vi "Read Mission Upload Msg.vi"(8 "error in (no error)":errorcluster, 11 "Load Mission Message in":refnum<class "Mission Upload Message.lvclass">) -> (0 "error out":errorcluster, 2 "Mission":T1[](array[typedef]) {"GPS Longitude" format="%.6g"; "GPS Latitude" format="%.6g"}, 3 "Load Mission Message out":refnum<class "Mission Upload Message.lvclass">)   [LabVIEW 2015, in "RDS Child Messages.lvlib" / "Mission Upload Message.lvclass"]
uses:
  Mission Upload Message.lvclass
  RDS Mission Controller Actor/MissionOp.ctl
  Mission Upload Message.lvclass/Mission Upload Message.ctl
  RDS Mission Controller Actor/RDS Mission Controller Actor.lvlib
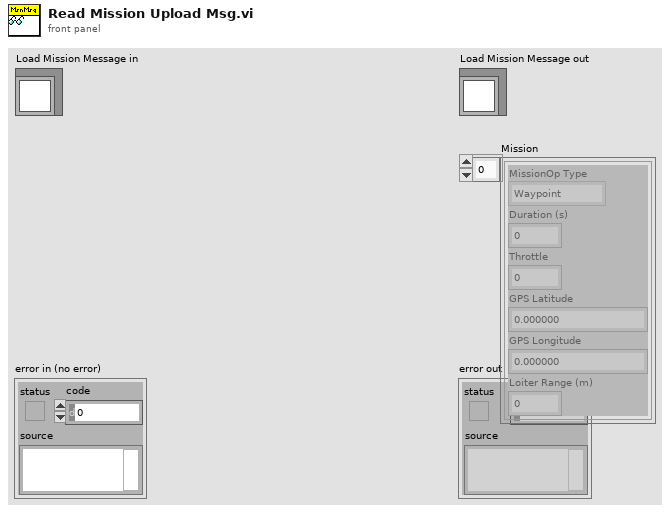
[diagram p1: front panel]
types:
  T1 = typedef "RDS Mission Controller Actor.lvlib/MissionOp.ctl" = cluster{"MissionOp Type":enum16{"Waypoint", "Loiter", "Wait", "Deploy AIP", "Stow AIP"}, "Duration (s)":u16, "Throttle":i16, "GPS Latitude":dbl, "GPS Longitude":dbl, "Loiter Range (m)":u16}
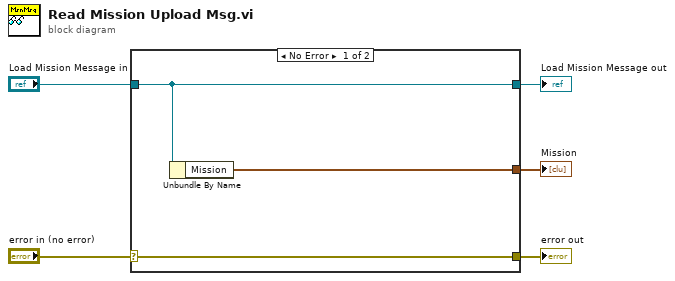
[diagram p0: block diagram]
diagram:
  n1 = case shown="No Error" "error in (no error)" {
    selector: "error in (no error)" -> [w8 w9]
    tunnel: [w8 w9] -> w4
    tunnel: [w7 w10] -> w2
    tunnel: "Load Mission Message in" -> [w7 w10]
    tunnel: [w6 _] -> w1
    frame No Error {
      n2 = Unbundle By Name(w7) -> ("Mission"=w6:T1[])
    }
    frame Error {
    }
  }
  "error out" <- w4
  "Load Mission Message out" <- w2
  "Mission" <- w1
